vi "GUI_OpticalSpectrometer.vi"() -> ()   [LabVIEW 2013]
panel:
  out "new Slow Data":bool
  out "new Device Data":bool
  in  "Tab Control":enum32{"Main", "Network settings", "internal"}(tab)
  out "array 2":dbl[](graph)=[-0.061346, -0.033825, -0.00088, -0.074669, -0.00201, -0.026885, -0.047095, -0.151322, -0.008371, 0.065125, 0.005817, -0.023408, 0.092676, 0.146426, 0.031995, 0.10524, 0.048758, 0.071596, 0.064967, 0.005247, -0.044093, -0.135153, -0.197466, -0.05307, -0.178929, -0.142798, -0.260601, -0.269352, -0.155307, -0.044906, -0.003241, 0.051496, 0.272465, 0.344122, 0.43635, 0.726556, 0.707702, 0.766922, 0.905498, 0.896567, 1.008759, 1.082142, 0.89412, 0.81031, 0.662588, 0.69242, 0.458403, 0.42714, 0.284239, 0.200704, -0.042121, -0.124136, -0.097584, -0.279723, -0.149904, -0.151625, -0.164074, -0.074535, -0.18067, -0.005619, -0.030632, -0.007923, -0.00569, 0.157924, 0.132593, 0.176677, 0.051413, 0.033802, -0.025755, -0.012477, 0.091722, -0.037117, -0.092774, -0.028783, -0.025598, -0.047595, -0.037073, -0.013775, 0.019461, 0.073427, 0.018275, -0.075507, -0.01765, 0.061887, 0.034105, -0.011361, 0.041433, 0.127522, -0.009118, -0.006842, -0.061769, -0.093199, 0.036108, -0.1247, 0.031183, -0.066401, -0.115517, -0.072946, -0.11326, 0.024127, 0.077506, 0.078651, -0.044754, -0.013325, -0.032215, 0.146745, 0.058399, 0.047647, 0.108466, 0.07484, 0.095157, -0.03767, -0.016345, 0.053104, -0.074904, 0.039642, -0.003835, 0.053729, -0.113306, -0.059684, -0.011519, 0.103576, 0.102395, 0.029519, 0.085877, 0.046904, -0.006382, 0.076213, 0.096201, 0.078133, -0.075872, -0.044221, 0.001434, -0.066755, -0.05701, 0.001366, 0.019859, 0.012545, -0.097979, -0.067019, 0.084456, -0.034377, 0.058015, 0.004913, 0.106627, 0.019982, -0.036441, 0.063597, 0.046667, 0.057833, 0.076003, -0.069381, -0.017155, -0.077432, -0.12436, 0.006415, -0.043024, 0.035844, -0.021059, 0.020196, -0.017899, -0.018124, 0.022979, -0.019183, 0.031563, 0.111704, -0.030725, -0.063522, -0.010931, -0.005552, -0.09674, -0.101343, 0.011818, -0.019371, -0.075836, -0.044542, -0.109565, -0.109436, -0.057505, 0.023722, 0.053348, 0.00861, -0.029861, 0.057824, 0.086824, -0.009295, 0.000118, -0.026367, -0.020188, -0.091992, 0.003958, 0.064911, -0.041005, -0.007375, -0.076431, -0.023656, -0.082537, -0.090322, -0.08626, 0.016279]
  in  "setTrigger":bool
  in  "String":string="setRunMode>>on"
  in  "send":bool
  in  "setSave":bool
  out "save":bool
  in  "setExposure":dbl=0.4
  out "exposure":dbl=0.1
  out "trigger":bool
  out "gain":dbl
  in  "setGain":dbl=4.0
  out "error message":string
  out "error":bool
  out "data out":string
  in  "local Port":u16=61540
  in  "Remote Host":string="192.168.10.182"
  in  "port or service name":u16=65535
  in  "timeout ms (100)":i32=500
  out "fast ID":refnum<k16>
  out "slow ID":refnum<k16>
  out "error out":errorcluster
  in  "Data String":string
  out "image connection ID":refnum<k5>
  out "data connection ID":refnum<k5>
  out "connections":variant[](array[variant])=[variant(refnum<k16> refnum), variant(refnum<k16> refnum), variant(refnum<k5> refnum), variant(refnum<k5> refnum)]
  out "image ID":string
  out "data ID":string
  in  "time to wait":i32=10
  in  "milliseconds to wait":u32=50
  in  "Data String 2":string
  out "device responds":string="Cam1>>setExposure>>0.400000>>command accepted"
  out "error out 2":errorcluster
  in  "stop":bool
  # "61525"
  # "65535"
  # "61533"
  # "localhost"
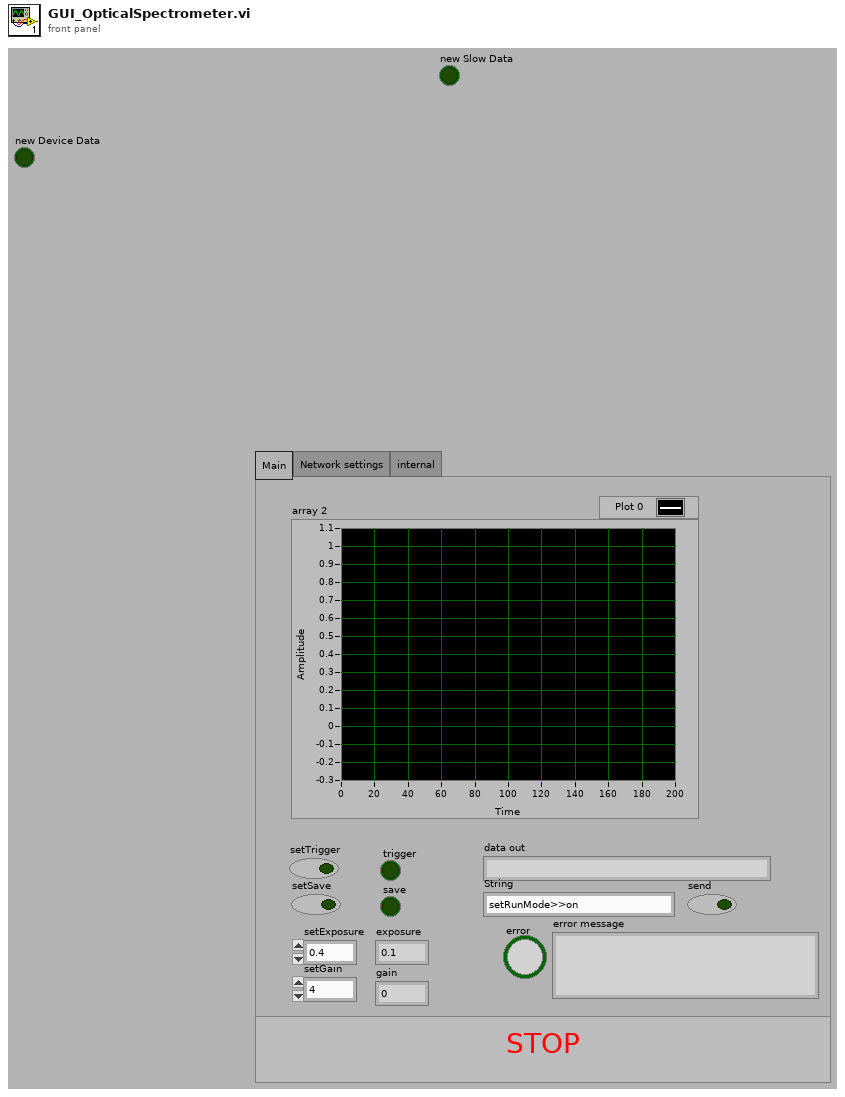
[diagram p1: front panel]
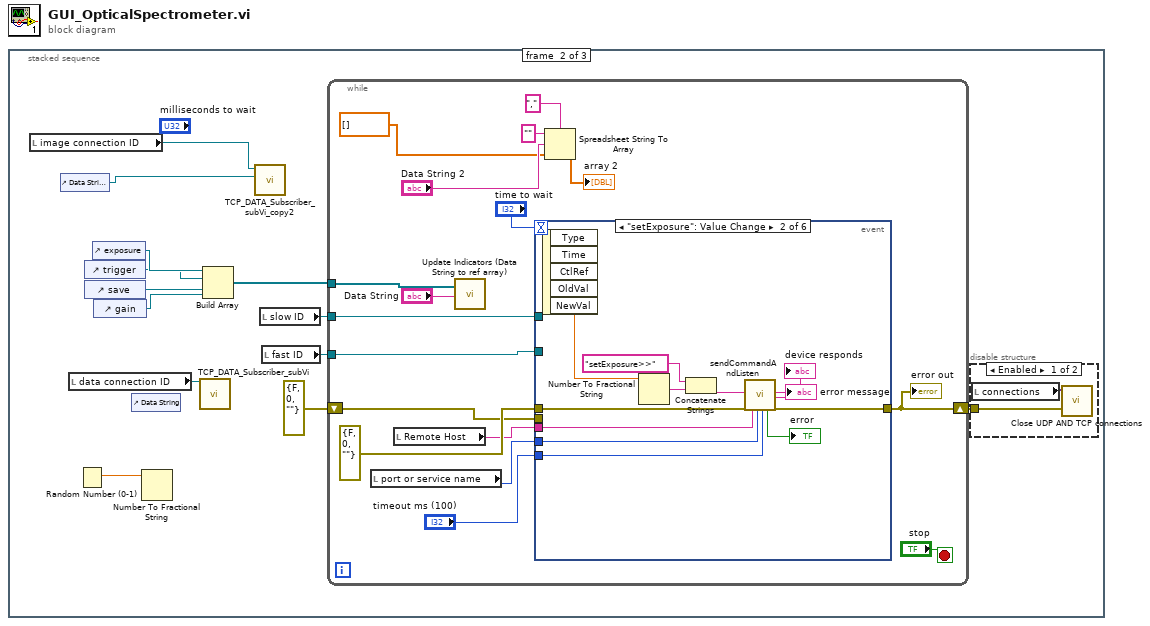
[diagram p0: block diagram]
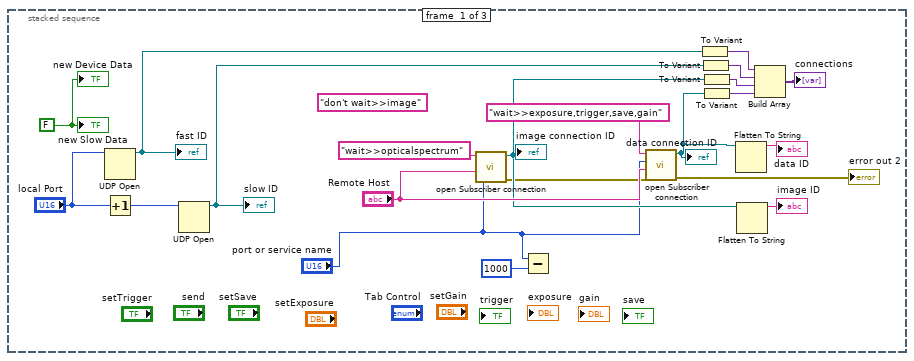
[diagram p2: hidden frame]
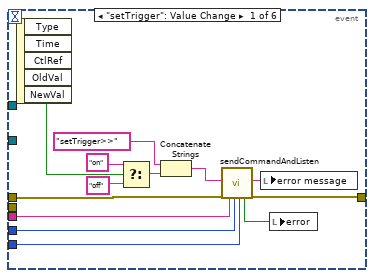
[diagram p4: hidden frame]
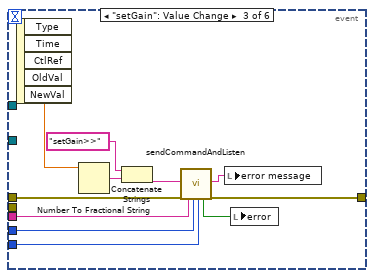
[diagram p5: hidden frame]
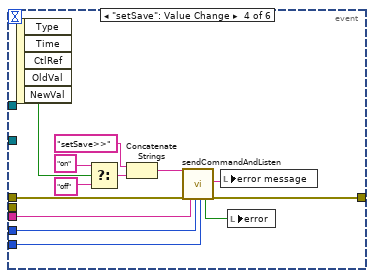
[diagram p6: hidden frame]
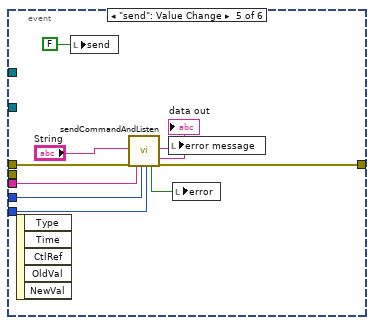
[diagram p7: hidden frame]
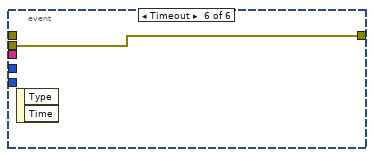
[diagram p8: hidden frame]
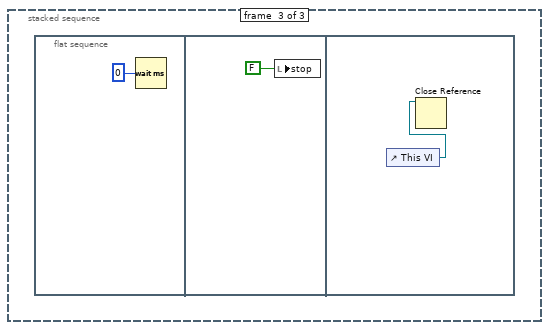
[diagram p9: hidden frame]
diagram:
  n1 = stacked-sequence {
    frame #0 {
      (unwired) "don't wait>>image" ("Subscriber list")
      w19 = FALSE ("new Device Data")
      n2 = UDP Open(11:"local Port") -> (port=w11:refnum<k16>)  [unwired: 4 in, 2 out]
      "fast ID" <- w11
      n3 = Increment(x="local Port") -> (x+1=w21:u16)
      n4 = UDP Open(11:w21) -> (port=w10:refnum<k16>)  [unwired: 4 in, 2 out]
      "slow ID" <- w10
      n5 = call "open Subscriber connection.vi"("Machine"="Remote Host", "Port"="port or service name", "Subscriber list"="wait>>opticalspectrum") -> ("error out"=w1:errorcluster, "connection ID"=w6:refnum<k5>)  [unwired: 3 in]
      "image connection ID" <- w6
      n6 = Subtract(x="port or service name", y=u16 1000) -> ()  [unwired: 1 out]
      n7 = call "open Subscriber connection.vi"("error in (no error)"=w1, "Machine"="Remote Host", "Port"="port or service name", "Subscriber list"="wait>>exposure,trigger,save,gain" ("Subscriber list 2")) -> ("error out"=→"error out 2":errorcluster, "connection ID"=w7:refnum<k5>)  [unwired: 2 in]
      "data connection ID" <- w7
      n8 = To Variant(anything=w11) -> (Variant=w9:variant)
      n9 = To Variant(anything=w10) -> (Variant=w8:variant)
      n10 = To Variant(anything=w6) -> (Variant=w14:variant)
      n11 = To Variant(anything=w7) -> (Variant=w13:variant)
      n12 = Flatten To String(anything=w7) -> (data string=→"data ID":string)  [unwired: 3 in, 2 out]
      n13 = Flatten To String(anything=w6) -> (data string=→"image ID":string)  [unwired: 3 in, 2 out]
      n14 = Build Array(w9, w8, w14, w13) -> (→"connections":variant[])
      "new Device Data" <- w19
      "new Slow Data" <- w19
    }
    frame #1 {
      n15 = local read "image connection ID"() -> (w23:refnum<k5>)
      n16 = control-ref of="Data String 2"() -> (w22:refnum<vi>)
      n17 = local read "data connection ID"() -> (w31:refnum<k5>)
      n18 = Random Number (0-1)() -> (number: 0 to 1=w25:dbl)
      n19 = control-ref of="trigger"() -> (w27:refnum<vi>)
      n20 = control-ref of="save"() -> (w28:refnum<vi>)
      n21 = control-ref of="exposure"() -> (w30:refnum<vi>)
      n22 = control-ref of="gain"() -> (w29:refnum<vi>)
      n23 = control-ref of="Data String"() -> ()  [unwired: 1 out]
      n24 = Number To Fractional String(number=w25) -> ()  [unwired: 3 in, 1 out]
      n25 = call "TCP_DATA_Subscriber_subVi.vi"("connection ID"=w31) -> ()  [unwired: 10 in, 1 out]
      n26 = Build Array(w30, w27, w28, w29) -> (w24:refnum<vi>[])
      n27 = call "TCP_DATA_Subscriber_subVi_copy2.vi"("data String"=w22, "connection ID"=w23) -> ()  [unwired: 9 in, 1 out]
      n28 = local read "slow ID"() -> (w32:refnum<k16>)
      n29 = local read "fast ID"() -> (w33:refnum<k16>)
      n30 = while {
        tunnel: w33 -> [w42]
        shift-right: [w47] -> w26
        shift-left: errorcluster {"status"=FALSE, "code"=0, "source"=""} ("error out") -> [w48]
        tunnel: w32 -> [w43]
        tunnel: w24 -> [w50]
        stop <- "stop" stop-if-true
        n31 = local read "port or service name"() -> (w44:u16)
        n32 = local read "Remote Host"() -> (w45:string)
        n33 = call "Update Indicators (Data String to ref array).vi"("Array"=w50, "Data String"="Data String") -> ()  [unwired: 12 in, 2 out]
        n34 = event shown="[1] \"setExposure\": Value Change" {
          selector: _ -> [_ _ _ _ _ _]
          dyn-events: _ -> [_ _ _ _ _ _]
          timeout: "time to wait" -> [_ _ _ _ _ _]
          tunnel: w42 -> [_ _ _ _ _ _]
          tunnel: [w56 w73 w84 w94 w109 w113] -> w47
          tunnel: errorcluster {"status"=FALSE, "code"=0, "source"=""} ("error out") -> [w57 w74 w85 w95 w110 _]
          tunnel: w45 -> [w59 w72 w83 w96 w108 _]
          tunnel: w44 -> [w60 w71 w82 w93 w107 _]
          tunnel: "timeout ms (100)" -> [w61 w70 w81 w92 w106 _]
          tunnel: w43 -> [_ _ _ _ _ _]
          tunnel: w48 -> [_ _ _ _ _ w113]
          event "setTrigger": Value Change {
            n35 = event-data() -> ("NewVal"=w66:bool)  [unwired: 1 in, 4 out]
            n36 = Select(t="on", s=w66, f="off") -> (s? t:f=w62:string)
            n37 = Concatenate Strings("setTrigger>>" ("data in"), w62) -> (w58:string)
            n38 = call "sendCommandAndListen.vi"("command in"=w58, "error in"=w57, "Remote Host"=w59, "port or service name"=w60, "timeout ms (100)"=w61) -> ("error"=w54:bool, "error message"=w55:string, "error out"=w56:errorcluster)  [unwired: 7 in, 5 out]
            n39 = local write "error message"(w55) -> ()
            n40 = local write "error"(w54) -> ()
          }
          event "setExposure": Value Change {
            n41 = event-data() -> ("NewVal"=w76:dbl)  [unwired: 1 in, 4 out]
            n42 = Number To Fractional String(number=w76) -> (F-format string=w77:string)  [unwired: 3 in]
            n43 = Concatenate Strings("setExposure>>" ("data in"), w77) -> (w75:string)
            n44 = call "sendCommandAndListen.vi"("command in"=w75, "error in"=w74, "Remote Host"=w72, "port or service name"=w71, "timeout ms (100)"=w70) -> ("error"=→"error":bool, "error message"=→"error message":string, "device responds"=→"device responds":string, "error out"=w73:errorcluster)  [unwired: 7 in, 4 out]
          }
          event "setGain": Value Change {
            n45 = event-data() -> ("NewVal"=w87:dbl)  [unwired: 1 in, 4 out]
            n46 = Number To Fractional String(number=w87) -> (F-format string=w88:string)  [unwired: 3 in]
            n47 = Concatenate Strings("setGain>>" ("data in"), w88) -> (w86:string)
            n48 = call "sendCommandAndListen.vi"("command in"=w86, "error in"=w85, "Remote Host"=w83, "port or service name"=w82, "timeout ms (100)"=w81) -> ("error"=w79:bool, "error message"=w80:string, "error out"=w84:errorcluster)  [unwired: 7 in, 5 out]
            n49 = local write "error message"(w80) -> ()
            n50 = local write "error"(w79) -> ()
          }
          event "setSave": Value Change {
            n51 = event-data() -> ("NewVal"=w102:bool)  [unwired: 1 in, 4 out]
            n52 = Select(t="on", s=w102, f="off") -> (s? t:f=w98:string)
            n53 = Concatenate Strings("setSave>>" ("data in"), w98) -> (w97:string)
            n54 = call "sendCommandAndListen.vi"("command in"=w97, "error in"=w95, "Remote Host"=w96, "port or service name"=w93, "timeout ms (100)"=w92) -> ("error"=w90:bool, "error message"=w91:string, "error out"=w94:errorcluster)  [unwired: 7 in, 5 out]
            n55 = local write "error message"(w91) -> ()
            n56 = local write "error"(w90) -> ()
          }
          event "send": Value Change {
            n57 = event-data() -> ()  [unwired: 1 in, 5 out]
            n58 = local write "send"(FALSE ("sent")) -> ()
            n59 = call "sendCommandAndListen.vi"("command in"="String", "error in"=w110, "Remote Host"=w108, "port or service name"=w107, "timeout ms (100)"=w106) -> ("error"=w104:bool, "error message"=w105:string, "data out"=→"data out":string, "error out"=w109:errorcluster)  [unwired: 7 in, 4 out]
            n60 = local write "error message"(w105) -> ()
            n61 = local write "error"(w104) -> ()
          }
          event Timeout {
            n62 = event-data() -> ()  [unwired: 1 in, 2 out]
          }
        }
        "error out" <- w47
        n63 = Spreadsheet String To Array(delimiter (Tab)=",", format string="", spreadsheet string="Data String 2", array type (2D Dbl)=dbl[] []) -> (array=→"array 2":dbl[])
      }
      n64 = disable-structure shown="Enabled" {
        disable-tunnel: w26 -> [w35 _]
        frame Enabled {
          n65 = local read "connections"() -> (w36:variant[])
          n66 = call "Close UDP AND TCP connections.vi"("error in"=w35, "appended array"=w36) -> ()  [unwired: 6 in]
        }
        frame Disabled {
        }
      }
    }
    frame #2 {
      n67 = flat-sequence {
        frame #0 {
          n68 = Wait (ms)(milliseconds to wait=u32 0) -> ()  [unwired: 1 out]
        }
        frame #1 {
          n69 = local write "stop"(FALSE ("stop")) -> ()
        }
        frame #2 {
          n70 = control-ref of="This VI"() -> (w116:refnum<vi>)
          n71 = Close Reference(reference=w116) -> ()  [unwired: 1 in, 1 out]
        }
      }
    }
  }
